vi "Set FIFO Names in IO Node.vi"(8 "error in (no error)":errorcluster, 10 "Array":string[](array[string]), 11 "Panel in":refnum<vi>) -> (0 "error out":errorcluster)   [LabVIEW 2014, in "SPI Engine Scripting.lvlib"]
doc: "Changes the value in the FIFO controls on the front panel of the new IO Node."
uses:
  SPI Engine Scripting.lvlib
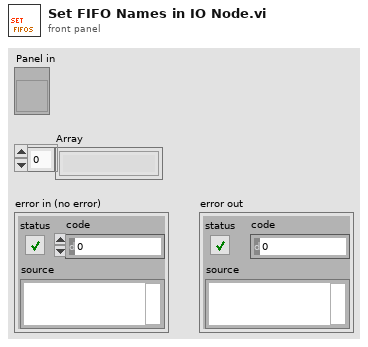
[diagram p1: front panel]
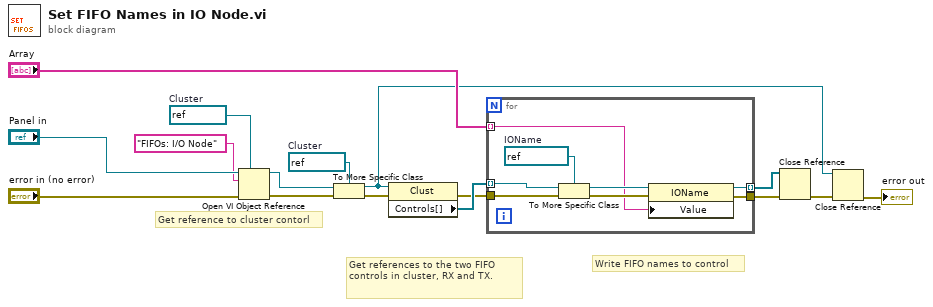
[diagram p0: block diagram]
diagram:
  w2 = refnum<vi> refnum  # Cluster
  w1 = refnum<vi> refnum  # Cluster
  # "Get references to the two FIFO controls in cluster, RX and TX."
  # "Write FIFO names to control"
  # "Get reference to cluster contorl"
  n1 = Open VI Object Reference(7:w1, 8:"error in (no error)", 10:"FIFOs: I/O Node" ("name/order"), 11:"Panel in") -> (0:w3:errorcluster, 3:w4:refnum<vi>)
  n2 = To More Specific Class(target class=w2, reference=w4, error in=w3) -> (specific class reference=w15:refnum<vi>, error out=w14:errorcluster)
  n3 = property class="Clust"(reference=w15, error in=w14) -> (error out=w9:errorcluster, "Controls[]"=w10:refnum<vi>[])  [unwired: 1 out]
  n4 = for {
    tunnel: [w24] -> w7 mode=indexing
    tunnel: [w23] -> w8
    tunnel: w9 -> [w19]
    tunnel: w10 -> [w18] mode=indexing
    tunnel: "Array" -> [w17] mode=indexing
    w20 = refnum<vi> refnum  # IOName
    n5 = To More Specific Class(target class=w20, reference=w18, error in=w19) -> (specific class reference=w21:refnum<vi>, error out=w22:errorcluster)
    n6 = property class="IOName"(reference=w21, error in=w22, "Value"=w17) -> (reference out=w24:refnum<vi>, error out=w23:errorcluster)
  }
  n7 = Close Reference(reference=w7, error in (no error)=w8) -> (error out=w6:errorcluster)
  n8 = Close Reference(reference=w15, error in (no error)=w6) -> (error out=→"error out":errorcluster)
